vi "LV9_4.vi"() -> ()   [LabVIEW 2011]
uses:
  <vilib>/imath/engines/lvmath2/RunTimeEngine/ErrorHandling/NIMS_Finalize Error.vi
  <vilib>/imath/engines/lvmath2/RunTimeEngine/NodeEndStatement/NIMS_NodeEndStatement_Output.vi
  <instcachedir>/0/NIMS_NodeEndStatement_Output_53EC0D466D134D7ABD903AC30B43404B.lvgen/NIMS_NodeEndStatement_Output_53EC0D466D134D7ABD903AC30B43404B_005.vi
  <instcachedir>/0/NIMS_NodeEndStatement_Output_53EC0D466D134D7ABD903AC30B43404B.lvgen/NIMS_NodeEndStatement_Output_53EC0D466D134D7ABD903AC30B43404B_002.vi
  <vilib>/imath/engines/lvmath2/RunTimeEngine/BuiltInFunctions/randnormal/NIMS_randnormal(Str,I32).vi
  <vilib>/imathl/engines/lvmath/Functions/Error Handling/Create Error.vi
  <vilib>/imath/engines/lvmath2/RunTimeEngine/BuiltInFunctions/randnormal/NIMS_randnormal(1,I32).vi
  <vilib>/imath/engines/lvmath2/RunTimeEngine/ArithmeticOperatorToken/NIMS_ArithmeticOperator_plus.vi
  <instcachedir>/0/NIMS_ArithmeticOperator_plus_1E95F7DAB906458CBECCADBE8E6FD739.lvgen/NIMS_ArithmeticOperator_plus_1E95F7DAB906458CBECCADBE8E6FD739_004.vi
  <vilib>/imath/engines/lvmath2/RunTimeEngine/ErrorHandling/NIMS_Create Error From Enums.vi
  <vilib>/imath/engines/lvmath2/RunTimeEngine/BuiltInFunctions/length/NIMS_length(GV).vi
  <instcachedir>/0/NIMS_length(GV)_08A3D13377FD4E4B96F5795FBF3698FA.lvgen/NIMS_length(GV)_08A3D13377FD4E4B96F5795FBF3698FA_000.vi
  <vilib>/imath/engines/lvmath2/RunTimeEngine/BuiltInFunctions/fft/NIMS_fft(GV).vi
  <instcachedir>/0/NIMS_fft(GV)_4C6467FC22F84E4BA42517A07EF978B0.lvgen/NIMS_fft(GV)_4C6467FC22F84E4BA42517A07EF978B0_000.vi
  <vilib>/imath/engines/lvmath2/RunTimeEngine/BuiltInFunctions/abs/NIMS_abs(signed).vi
  <instcachedir>/0/NIMS_abs(signed)_C4FCB8E6058B49B797C7C8D53CA5F6EC.lvgen/NIMS_abs(signed)_C4FCB8E6058B49B797C7C8D53CA5F6EC_006.vi
  <vilib>/imath/engines/lvmath2/RunTimeEngine/ErrorHandling/NIMS_Error From Error Code.vi
  <vilib>/imath/engines/lvmath2/RunTimeEngine/BuiltInFunctions/ifft2d/NIMS_ifft2d.vi
  <vilib>/imath/engines/lvmath2/RunTimeEngine/RangeToken/NIMS_Range.vi
  <instcachedir>/0/NIMS_Range_0B7635FB69F84E19AA68E7FF959DF37C.lvgen/NIMS_Range_0B7635FB69F84E19AA68E7FF959DF37C_001.vi
  <vilib>/imath/engines/lvmath2/RunTimeEngine/VariableToken/Read/NIMS_Get Elements - SorM(_) - Check(_).vi
  <instcachedir>/0/NIMS_Get Elements - SorM(_) - Check(_)_561A7B7910804DA3BBA41B7F4E44AAB4.lvgen/NIMS_Get Elements - SorM(_) - Check(_)_561A7B7910804DA3BBA41B7F4E44AAB4_008.vi
  <instcachedir>/0/NIMS_Range_0B7635FB69F84E19AA68E7FF959DF37C.lvgen/NIMS_Range_0B7635FB69F84E19AA68E7FF959DF37C_000.vi
panel:
  in  "stop":bool
  in  "Noise level":dbl(slide) step=0.001 scale=0.0..2.0
  out "Signal":cluster{"TA":dbl[], "A":dbl[]}(graph)
  in  "Period":dbl(slide) step=0.001 scale=0.002..0.008
  out "Autocorrelation":cluster{"TA":dbl[], "A":dbl[]}(graph)
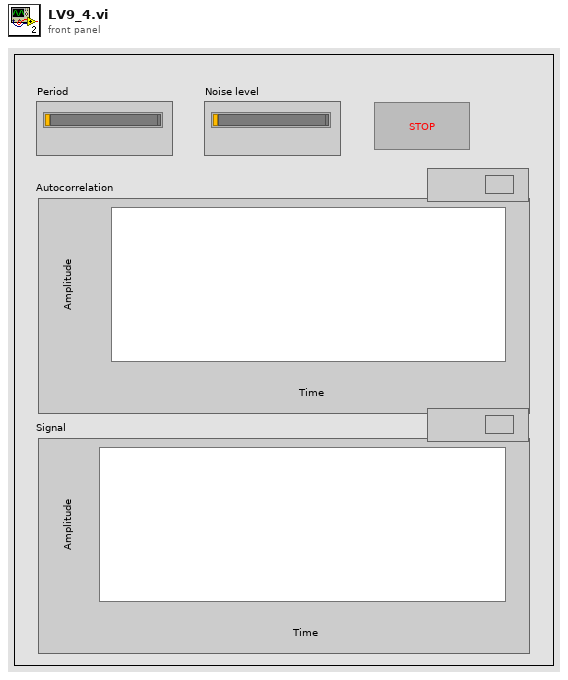
[diagram p1: front panel]
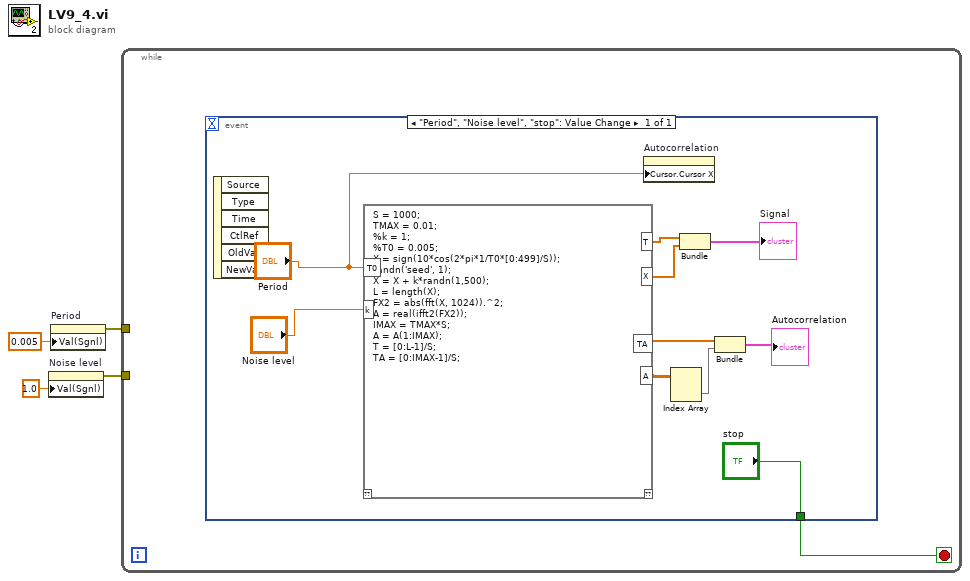
[diagram p0: block diagram]
diagram:
  n1 = property on="Noise level" class="Slide (strict)"("Val(Sgnl)"=1.0 ("Value (Signaling)")) -> (error out=w3:errorcluster)  [unwired: 2 in, 1 out]
  n2 = property on="Period" class="Slide (strict)"("Val(Sgnl)"=0.005 ("Value (Signaling)")) -> (error out=w4:errorcluster)  [unwired: 2 in, 1 out]
  n3 = while {
    tunnel: w4 -> [_]
    tunnel: w3 -> [_]
    stop <- w5 stop-if-true
    n4 = event shown="[0] \"Period\", \"Noise level\", \"stop\": Value Change" {
      selector: _ -> [_]
      dyn-events: _ -> [_]
      timeout: _ -> [_]
      tunnel: ["stop"] -> w5
      event "Period", "Noise level", "stop": Value Change {
        n5 = event-data() -> ()  [unwired: 1 in, 6 out]
        n6 = mathscript code="S = 1000;\nTMAX = 0.01;\n%k = 1;\n%T0 = 0.005;\nX = sign(10*cos(2*pi*1/T0*[0:499]/S));\nrandn('seed', 1);\nX = X + k*randn(1,500);\nL = length(X);\nFX2 = abs(fft(X, 1024)).^2;\nA = real(ifft2(FX2));\nIMAX = TMAX*S;\nA = A(1:IMAX);\nT = [0:L-1]/S;\nTA = [0:IMAX-1]/S;"("T0"="Period", "k"="Noise level") -> ("A"=w12:dbl[][], "TA"=w13:dbl[], "T"=w15:dbl[], "X"=w14:dbl[])  [unwired: 1 in, 1 out]
        n7 = property on="Autocorrelation" class="XYGraph (strict)"("Cursor.Cursor X"="Period") -> ()  [unwired: 2 in, 2 out]
        n8 = Index Array(array=w12) -> (element=w11:dbl[])  [unwired: 2 in]
        n9 = Bundle("T"=w15, "X"=w14) -> (→"Signal":cluster{"T":dbl[], "X":dbl[]})  [unwired: 1 in]
        n10 = Bundle("TA"=w13, "A"=w11) -> (→"Autocorrelation":cluster{"TA":dbl[], "A":dbl[]})  [unwired: 1 in]
      }
    }
  }
